vi "DAQs.vi"(0 "sample channels":tag, 1 "rate":dbl, 5 "gain channels":tag, 7 "Sync or not":bool, 9 "Counter":tag="Dev1/ctr0", 11 "Ttrigger channels":tag="/Dev1/PFI12", 13 "Frequency":dbl=1.0 format="%.6f") -> (3 "gain task":refnum<k21>, 4 "sample task":refnum<k21>, 6 "task out":refnum<k21>, 10 "SampClk.Rate 2":dbl, 14 "Actual Frequency":dbl, 15 "error out":errorcluster)   [LabVIEW 2016]
uses:
  <vilib>/DAQmx/create/channels.llb/DAQmx Create Channel (AO-Voltage-Basic).vi
  <vilib>/DAQmx/create/channels.llb/DAQmx Create Channel (AI-Voltage-Basic).vi
  <vilib>/DAQmx/configure/timing.llb/DAQmx Timing (Sample Clock).vi
  <vilib>/DAQmx/create/channels.llb/DAQmx Create Channel (CO-Pulse Generation-Frequency).vi
  <vilib>/DAQmx/configure/timing.llb/DAQmx Timing (Implicit).vi
  <vilib>/DAQmx/configure/trigger.llb/DAQmx Start Trigger (Digital Edge).vi
  <resource>/objmgr/daqmx.rc
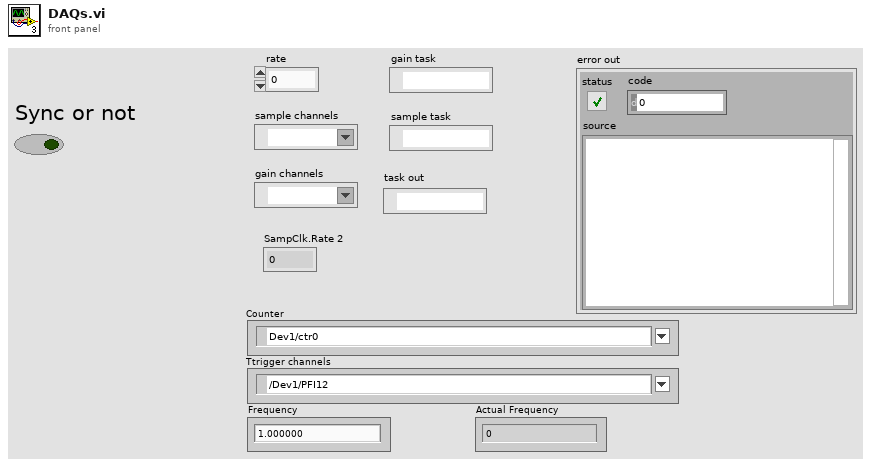
[diagram p1: front panel]
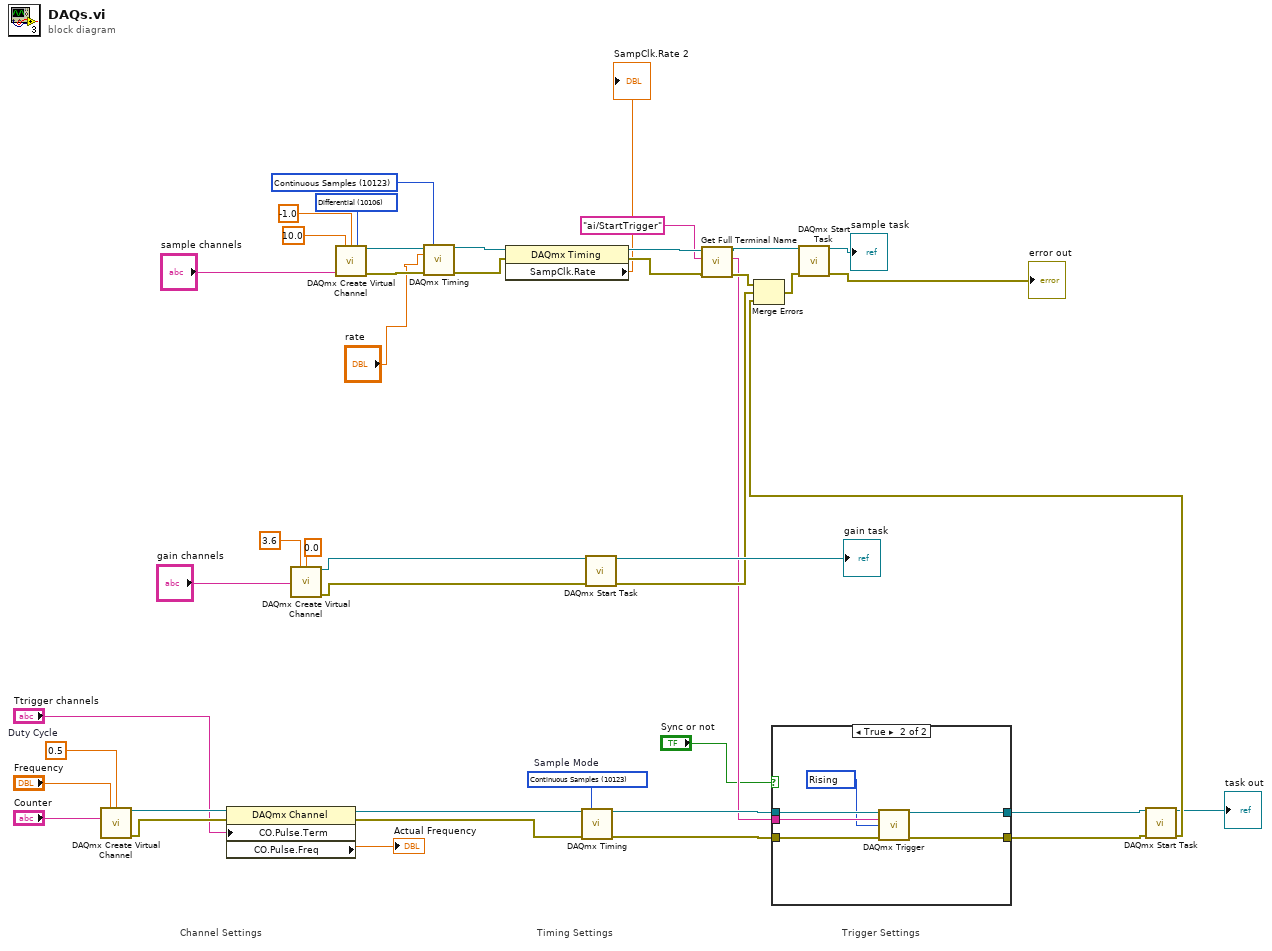
[diagram p0: block diagram]
diagram:
  w7 = 0.5  # Duty Cycle
  w19 = 10123 items=["Finite Samples"=10178, "Continuous Samples"=10123, "Hardware Timed Single Point"=12522]  # Sample Mode
  w33 = 10106 items=["default"=-1, "RSE"=10083, "NRSE"=10078, "Differential"=10106, "Pseudodifferential"=12529] ("input terminal configuration")
  w24 = 10123 items=["Finite Samples"=10178, "Continuous Samples"=10123, "Hardware Timed Single Point"=12522] ("sample mode")
  # "Trigger Settings"
  # "Timing Settings"
  # "Channel Settings"
  n1 = call-poly <vilib>:"DAQmx Create Virtual Channel.vi"("frequency"="Frequency", "duty cycle"=w7, "counter"="Counter") -> ("task out"=w13:refnum<k21>, "error out"=w12:errorcluster)  [unwired: 11 in]
  n2 = property class="DAQmx Channel"(reference=w13, error in=w12, "CO.Pulse.Term"="Ttrigger channels") -> (reference out=w9:refnum<k21>, error out=w10:errorcluster, "CO.Pulse.Freq"=→"Actual Frequency":dbl)
  n3 = call-poly <vilib>:"DAQmx Create Virtual Channel.vi"("maximum value"=3.6, "minimum value"=0.0, "physical channels"="gain channels") -> ("task out"=w23:refnum<k21>, "error out"=w21:errorcluster)  [unwired: 11 in]
  n4 = call-poly <vilib>:"DAQmx Create Virtual Channel.vi"("maximum value"=10.0, "minimum value"=-1.0, "input terminal configuration"=w33, "physical channels"="sample channels") -> ("task out"=w28:refnum<k21>, "error out"=w27:errorcluster)  [unwired: 10 in]
  n5 = call-poly <vilib>:"DAQmx Timing.vi"("task/channels in"=w28, "sample mode"=w24, "rate"="rate", "error in"=w27) -> ("task out"=w30:refnum<k21>, "error out"=w34:errorcluster)  [unwired: 10 in]
  n6 = property class="DAQmx Timing"(reference=w30, error in=w34) -> (reference out=w41:refnum<k21>, error out=w40:errorcluster, "SampClk.Rate"=→"SampClk.Rate 2":dbl)
  n7 = call-poly <vilib>:"DAQmx Timing.vi"("task/channels in"=w9, "sample mode"=w19, "error in"=w10) -> ("task out"=w17:refnum<k21>, "error out"=w16:errorcluster)  [unwired: 11 in]
  n8 = call <vilib>:"DAQmx Start Task.vi"("task/channels in"=w23, "error in"=w21) -> ("task out"=→"gain task":refnum<k21>, "error out"=w20:errorcluster)  [unwired: 12 in]
  n9 = call "Get Full Terminal Name.vi"("error in"=w40, "Local Terminal Name"="ai/StartTrigger" ("terminal"), "task/channels in"=w41) -> ("error out"=w39:errorcluster, "Terminal Name with Device Prefix"=w5:tag, "task out"=w37:refnum<k21>)  [unwired: 6 in]
  n10 = case shown="True" "Sync or not" {
    tunnel: w17 -> [w46 w52]
    tunnel: w16 -> [w45 w51]
    tunnel: [w45 w50] -> w15
    tunnel: [w46 w49] -> w14
    tunnel: w5 -> [_ w48]
    frame False {
    }
    frame True {
      w47 = 10280 items=["Rising"=10280, "Falling"=10171] ("edge")
      n11 = call-poly <vilib>:"DAQmx Trigger.vi"("task/channels in"=w52, "source"=w48, "edge"=w47, "error in"=w51) -> ("task out"=w49:refnum<k21>, "error out"=w50:errorcluster)  [unwired: 10 in]
    }
  }
  n12 = call <vilib>:"DAQmx Start Task.vi"("task/channels in"=w14, "error in"=w15) -> ("task out"=→"task out":refnum<k21>, "error out"=w4:errorcluster)  [unwired: 12 in]
  n13 = Merge Errors(w39, w20, w4) -> (w35:errorcluster)
  n14 = call <vilib>:"DAQmx Start Task.vi"("task/channels in"=w37, "error in"=w35) -> ("task out"=→"sample task":refnum<k21>, "error out"=→"error out":errorcluster)  [unwired: 12 in]
